vi "Write Mods.vi"(6 "Mods":cluster{"Double Click":bool, "Menu Key":bool}, 11 "Handle Mouse Down Msg in":refnum<class "Handle Mouse Down Msg.lvclass">) -> (3 "Handle Mouse Down Msg out":refnum<class "Handle Mouse Down Msg.lvclass">)   [LabVIEW 2017, in "Handle Mouse Down Msg.lvclass"]
uses:
  <vilib>/gpm_packages/@cs/Test-executive-builder/Source/Test Executive Builder View/Test Executive Builder View Messages/Handle Mouse Down Msg/Handle Mouse Down Msg.lvclass
  <vilib>/gpm_packages/@cs/Test-executive-builder/Source/Test Executive Builder View/Test Executive Builder View Messages/Handle Mouse Down Msg/Handle Mouse Down Msg.lvclass/Handle Mouse Down Msg.ctl
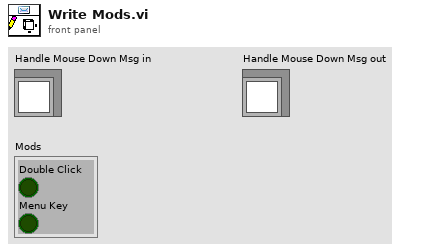
[diagram p1: front panel]
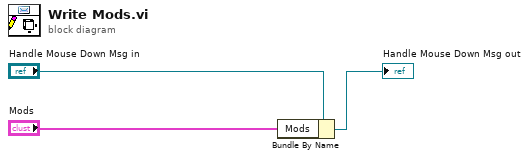
[diagram p0: block diagram]
diagram:
  n1 = Bundle By Name(cluster="Handle Mouse Down Msg in", "Mods"="Mods") -> (→"Handle Mouse Down Msg out":refnum<class "Handle Mouse Down Msg.lvclass">)
